vi "Transform to Rotation Matrix.vi"(1 "transform":T1) -> (0 "rotation matrix":T1)   [LabVIEW 2017, in "NI_Kinematics.lvlib"]
doc: "Returns the corresponding <B>rotation matrix</B> for the homogenous transform you specify.\n\n<B>.m file:</B> t2r"
uses:
  <vilib>/robotics/Kinematics/NI_Kinematics.lvlib
  <vilib>/Analysis/Matrix/Datatypes/RealMatrix.ctl
  <vilib>/Analysis/Matrix/NI_Matrix.lvlib
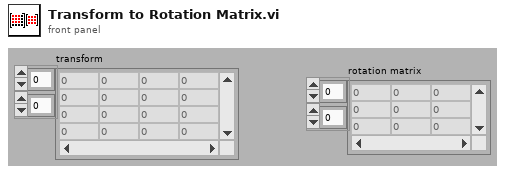
[diagram p1: front panel]
types:
  T1 = typedef "NI_Matrix.lvlib/RealMatrix.ctl" = dbl[][]
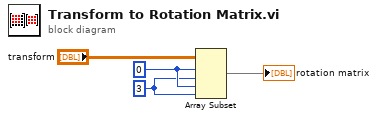
[diagram p0: block diagram]
diagram:
  w2 = 3 ("length")
  w3 = 0 ("index")
  n1 = Array Subset(array="transform", index (row)=w3, length (row)=w2, index (col)=w3, length (col)=w2) -> (→"rotation matrix":T1)
